vi "Get Channels Test.vi"() -> ()   [LabVIEW 2015, in "User Control Module Test.lvlib"]
uses:
  User Control Module Test.lvlib
  module/configuration/user control module configuration.lvclass
panel:
  out "x = y?":bool
  out "error out":errorcluster
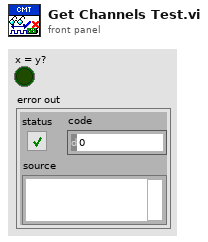
[diagram p1: front panel]
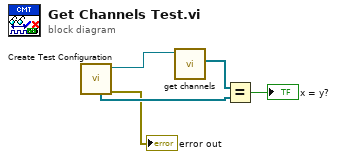
[diagram p0: block diagram]
diagram:
  n1 = call "Create Test Configuration.vi"() -> ("error out"=→"error out":errorcluster, "Module"=w5:refnum<class "user control module configuration.lvclass">, "Channels"=w3:refnum<class "TBM channel.lvclass">[])  [unwired: 6 in, 3 out]
  n2 = call-dynamic "get channels.vi"("fixed channel configuration in"=w5) -> ("channels"=w4:refnum<class "TBM channel.lvclass">[])  [unwired: 9 in, 1 out]
  n3 = Equal?(x=w4, y=w3) -> (x = y?=→"x = y?":bool)
